vi "MongoDB.SimpleExample2.vi"() -> ()   [LabVIEW 2014]
uses:
  Controls/Doc_TypeDef.ctl
  MongoDB.Collection.lvclass
  MongoDB.Client.lvclass
  MongoDB.Database.lvclass
panel:
  out "Cluster":T1={"String"="Test_ID", "I64"=0, "Bool"=TRUE, "Dbl_Array"=[0.04208234054769622, 0.6159072284708795, 0.9924706583884045, 0.9095839330222035, 0.884106028480875, 0.015388394824913165, 0.3936844840957101, 0.5660150245093465, 0.1650540886726075, 0.8706253940383701, 0.5192083162099523, 0.3985769664700203, 0.2732768418255602, 0.571749583229201, 0.69184633515106, 0.04043137440039146, 0.3832122802104301, 0.21648330177989594, 0.3975461276466077, 0.3225081050877523, 0.07348004479829107, 0.1793466173774676, 0.6140878844303679, 0.5463083733687983, 0.4995495694660945, 0.9914676953117344, 0.8547739160177218, 0.7991640317830502, 0.628953882592344, 0.15719094668429245, 0.6719434050298603, 0.1738587637177733, 0.991229086814548, 0.16493618776387975, 0.7872501917071991, 0.4103215352085412, 0.869897532002972, 0.48026601779022293, 0.3140688758805521, 0.6776368728429185, 0.17737760100880529, 0.27510758602931995, 0.6819654447011496, 0.960759533751685, 0.4313507815422317, 0.03725470116601115, 0.25754302581215294, 0.22441897627982832, 0.9336426404339386, 0.9080191203537264]}
  in  "error in (no error)":errorcluster
  out "error out":errorcluster
  out "Result":string="{ \"_id\" : ObjectId(\"550c366be59f891f54ed0277\"), \"String\" : \"Test_ID\", \"I64\" : 0, \"Bool\" : true, \"Dbl_Array\" : [0.042082340547696218, 0.61590722847087953, 0.99247065838840454, 0.90958393302220353, 0.884106028480875, 0.015388394824913165, 0.39368448409571011, 0.56601502450934649, 0.16505408867260751, 0.87062539403837014, 0.51920831620995234, 0.39857696647002028, 0.27327684182556022, 0.571749583229201, 0.69184633515106, 0.040431374400391462, 0.38321228021043008, 0.21648330177989594, 0.39754612764660768, 0.32250810508775229, 0.073480044798291066, 0.1793466173774676, 0.61408788443036788, 0.54630837336879834, 0.49954956946609452, 0.9914676953117344, 0.85477391601772179, 0.79916403178305018, 0.628953882592344, 0.15719094668429245, 0.67194340502986027, 0.17385876371777331, 0.991229086814548, 0.16493618776387975, 0.78725019170719912, 0.4103215352085412, 0.869897532002972, 0.48026601779022293, 0.3140688758805521, 0.67763687284291851, 0.17737760100880529, 0.27510758602931995, 0.68196544470114961, 0.960759533751685, 0.43135078154223172, 0.03725470116601115, 0.25754302581215294, 0.22441897627982832, 0.93364264043393863, 0.90801912035372645] }"
  in  "collectionName":string="testcollection1"
  in  "databaseName":string="labview_test"
  in  "connectionString":string="mongodb://labview_user:labview@ds045031.mongolab.com:45031/labview_test"
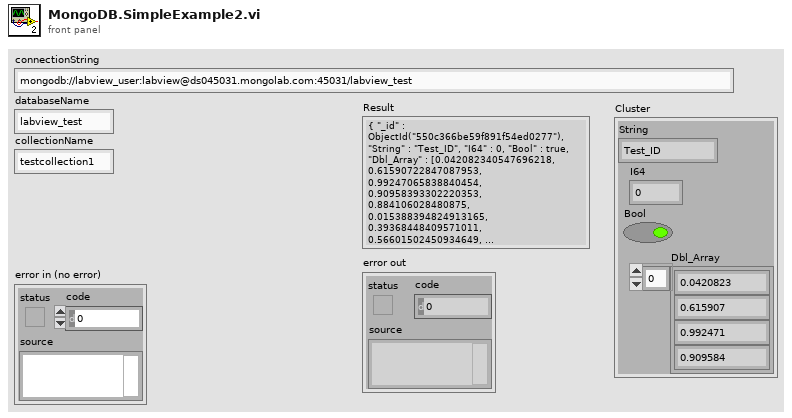
[diagram p1: front panel]
types:
  T1 = typedef "Doc_TypeDef.ctl" = cluster{"String":string, "I64":i64, "Bool":bool, "Dbl_Array":dbl[]}
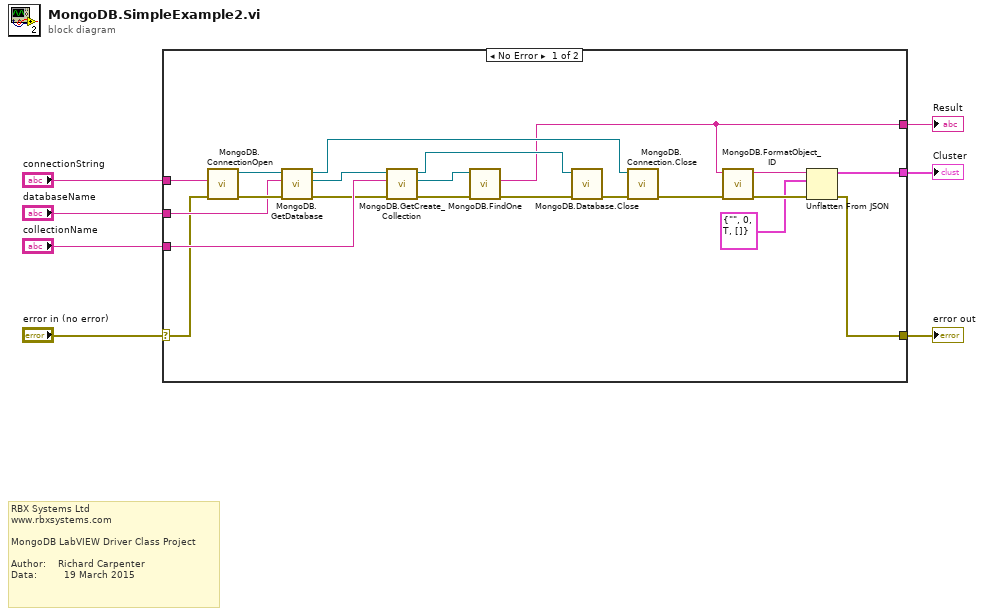
[diagram p0: block diagram]
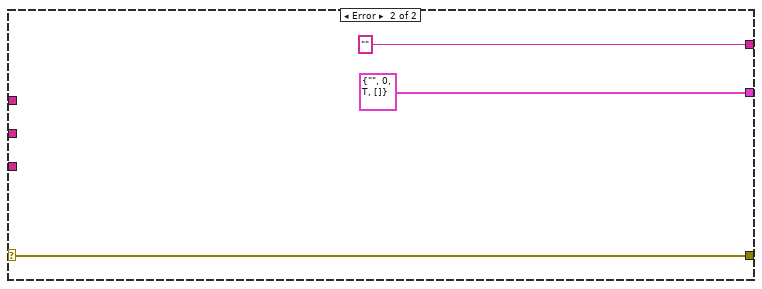
[diagram p2: hidden frame]
diagram:
  # "RBX Systems Ltd\nwww.rbxsystems.com\n\nMongoDB LabVIEW Driver Class Project\n\nAuthor:    Richard Carpenter\nData:         19 March 2015"
  n1 = case shown="No Error" "error in (no error)" {
    selector: "error in (no error)" -> [w15 w30]
    tunnel: "databaseName" -> [w26 _]
    tunnel: "connectionString" -> [w25 _]
    tunnel: "collectionName" -> [w23 _]
    tunnel: [w10 "" ("Result")] -> w4
    tunnel: [w13 w30] -> w3
    tunnel: [w14 T1 {"String"="", "I64"=0, "Bool"=TRUE, "Dbl_Array"=[]} ("Cluster")] -> w1
    frame No Error {
      n2 = call "MongoDB.ConnectionOpen.vi"("error in (no error)"=w15, "connectionString"=w25) -> ("error out"=w27:errorcluster, "MongoDB out"=w28:refnum<class "MongoDB.Client.lvclass">)  [unwired: 8 in]
      n3 = call "MongoDB.GetDatabase.vi"("error in (no error)"=w27, "databaseName"=w26, "MongoDB.Connection in"=w28) -> ("error out"=w22:errorcluster, "MongoDB.Database out"=w24:refnum<class "MongoDB.Database.lvclass">, "MongoDB.Connection out"=w21:refnum<class "MongoDB.Client.lvclass">)  [unwired: 6 in]
      n4 = call "MongoDB.GetCreate_Collection.vi"("error in (no error)"=w22, "collectionName"=w23, "MongoDB.Database in"=w24) -> ("error out"=w17:errorcluster, "MongoDB.Collection out"=w18:refnum<class "MongoDB.Collection.lvclass">, "MongoDB.Database out"=w19:refnum<class "MongoDB.Database.lvclass">)  [unwired: 6 in]
      n5 = call-dynamic "MongoDB.FindOne.vi"("error in (no error)"=w17, "MongoDB.Collection in"=w18) -> ("error out"=w16:errorcluster, "Result"=w10:string)  [unwired: 7 in, 1 out]
      n6 = call "MongoDB.Database.Close.vi"("error in (no error)"=w16, "MongoDB.Database in"=w19) -> ("error out"=w20:errorcluster)  [unwired: 9 in]
      n7 = call "MongoDB.Connection.Close.vi"("error in (no error)"=w20, "MongoDB in"=w21) -> ("error out"=w12:errorcluster)  [unwired: 9 in]
      n8 = call "MongoDB.FormatObject_ID.vi"("Error In"=w12, "JSON In"=w10) -> ("Error Out"=w11:errorcluster, "JSON Out"=w9:string)  [unwired: 8 in]
      n9 = Unflatten From JSON(JSON string=w9, type and defaults=T1 {"String"="", "I64"=0, "Bool"=TRUE, "Dbl_Array"=[]} ("Cluster"), error in (no error)=w11) -> (value=w14:T1, error out=w13:errorcluster)  [unwired: 4 in]
    }
    frame Error {
    }
  }
  "Result" <- w4
  "error out" <- w3
  "Cluster" <- w1
